vi "DAQMan TCP Data Stream.vi"() -> ()   [LabVIEW 2012]
uses:
  <userlib>/STM/_SubVIs/stm_MetaDataElement.ctl
  <userlib>/STM/TCP/stm_TCP Read Options.ctl
  Common/Controls/Waveform Header.ctl
  Common/Controls/Modified Waveform.ctl
  <userlib>/STM/TCP/STM Read Meta Data (TCP Ref).vi
  <userlib>/STM/TCP/STM Get Connection Reference (TCP).vi
  <userlib>/STM/TCP/STM Read Message (TCP).vi
panel:
  in  "Tab Control":enum32{"Wfm", "Modbus Wfm"}(tab)
  out "Acquired Data":sgl[][](graph)
  out "BlockID":u32
  out "size(s)":i32[](array[numeric])
  out "attributes (str)":string[][](array[string])
  out "Hdr Update Time":timestamp
  out "Acquired Data 2":sgl[][](graph)
  out "size(s) 2":i32[](array[numeric])
  out "BlockID 2":u32
  out "Hdr Update Time":timestamp
  out "attributes (str) 2":string[][](array[string])
  in  "Port":u16=5556
  in  "Name":T1="cDAQ1"
  out "Meta data":T1[](array[typedef])
  out "Updates":i32=2
  in  "client stop":bool
  in  "Target IP Address":string="localhost"
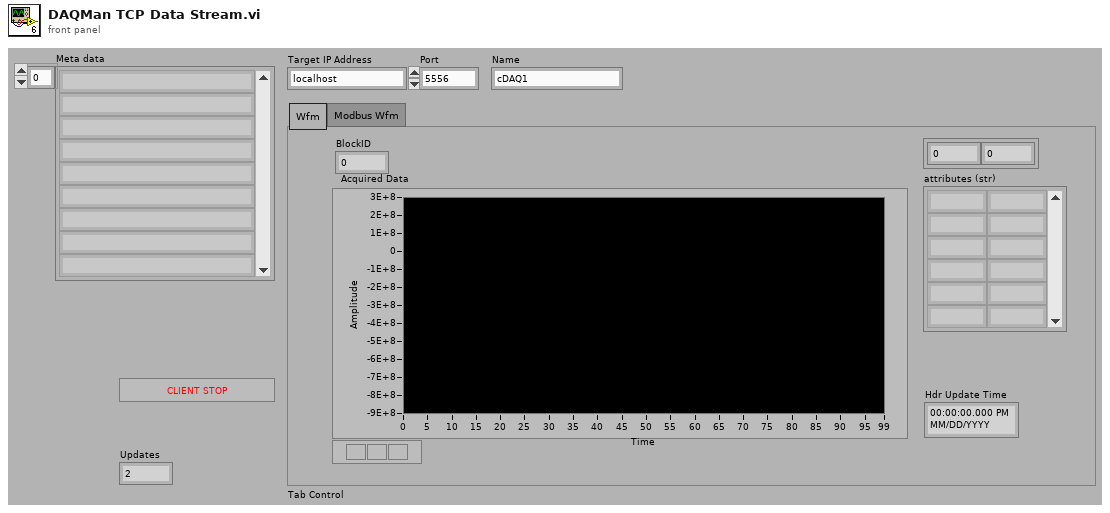
[diagram p1: front panel]
types:
  T1 = typedef "stm_MetaDataElement.ctl" = string
  T2 = typedef "stm_TCP Connection Info.ctl" = cluster{"connection ID":refnum<k5>, "Meta data":T1[]}
  T3 = typedef "stm_TCP Read Options.ctl" = cluster{"Ignore Timeout Error":bool, "timeout ms (1000)":i32}
  T4 = typedef "Waveform Header.ctl" = cluster{"dt":dbl, "attributes (str)":string[][]}
  T5 = enum16{"big-endian, network order", "native, host order", "little-endian"}
  T6 = typedef "Modified Waveform.ctl" = cluster{"BlockID":u32, "to (s)":dbl, "Y":sgl[][]}
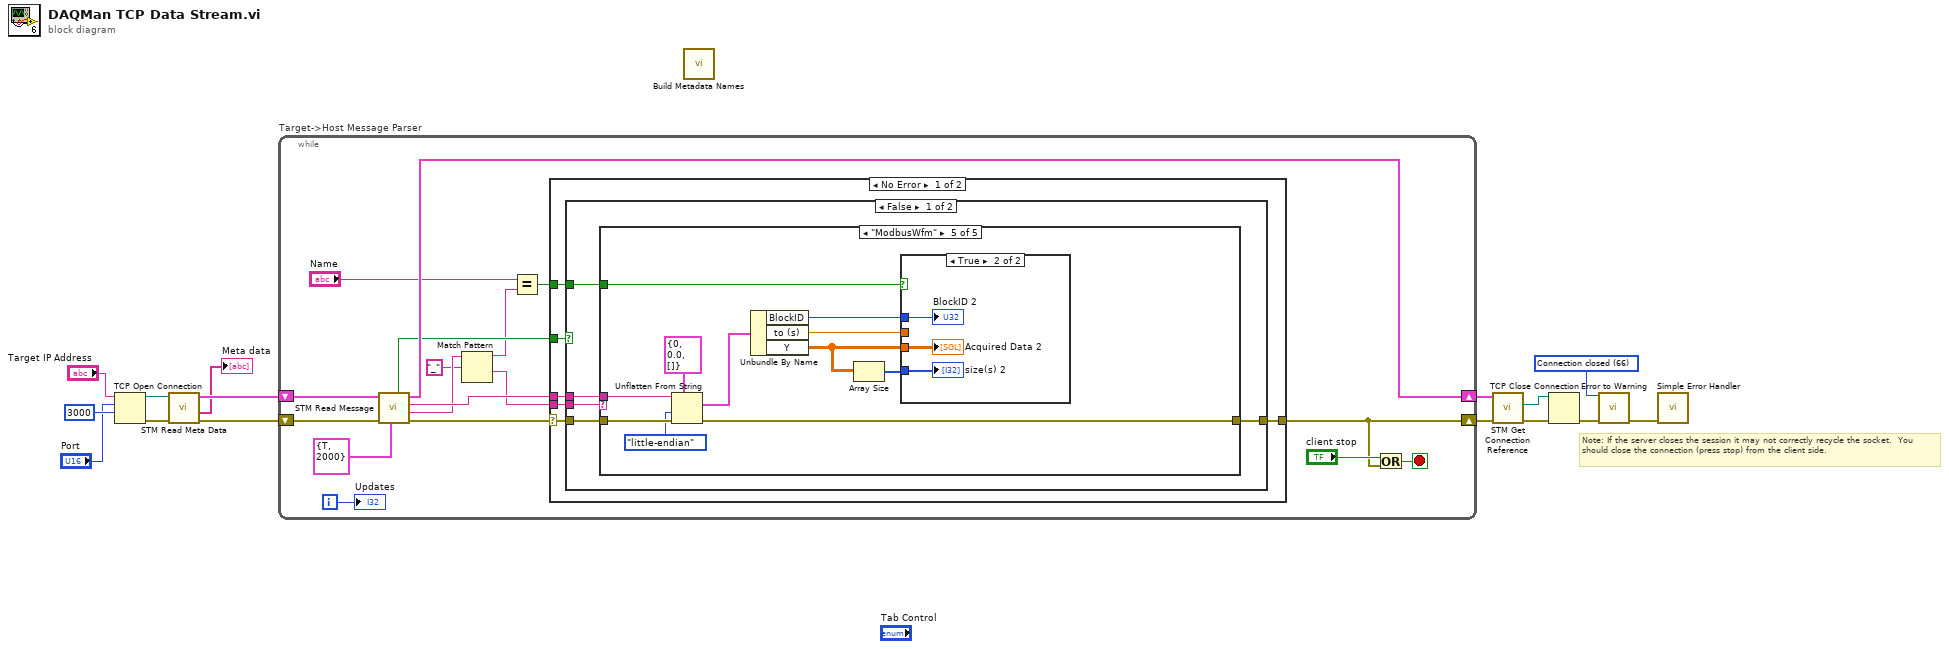
[diagram p0: block diagram]
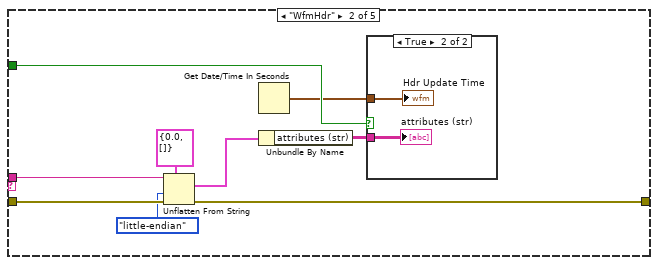
[diagram p3: hidden frame]
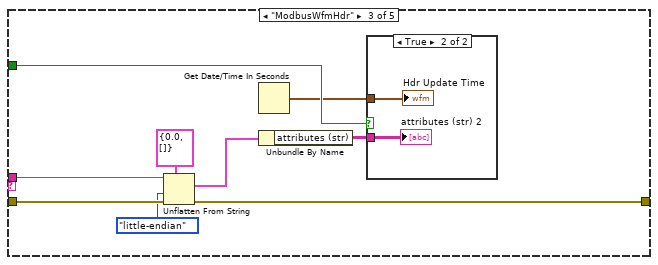
[diagram p5: hidden frame]
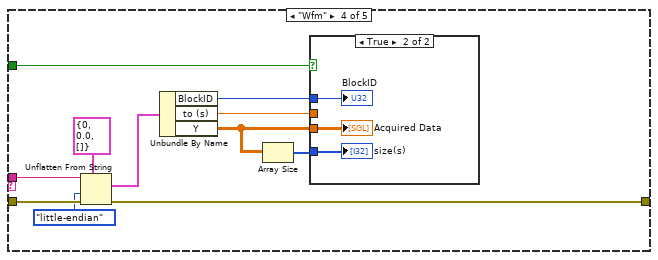
[diagram p7: hidden frame]
diagram:
  w12 = 66 items=["No Error", "Argument Error", "Memory Full", "Out of Zone", "End of File", "File Already Open", "Generic File IO Error", "File Not Found", "File Permission Error", "Disk Full", "Duplicate Path", "Too Many Files Open", "Not Enabled", "Resource File Not Found", "Cannot Add Resource", "Resource Not Found", "Image Not Found", "Image Memory Error", "Pen Does Not Exist", "Config Bad Type", "Config Token Not Found", "Config Parse Error", "Config Memory Error", "Bad External Code Format", "Bad External Code Offset", "External Code Not Present", "Null Window", "Destroy Window Mixup", "Null Menu", "Print Aborted", "Bad Print Record", "Print Driver Error", "Windows Error During Print", "Memory Error During Print", "Print Dialog Error", "Generic Print Error", "Invalid Device Refnum", "Device Not Found", "Device Parameter Error", "Device Unit Error", "Can't Open Device", "Device Call Aborted", "Generic Error", "Cancelled By User", "Object ID Too Low", "Object ID Too High", "Object Not In Heap", "Unknown Heap", "Bad DefProc ID", "DefProc Not In Table", "Message Out Of Range", "Null Method", "Unknown Message", "Manager Call Not Supported", "Bad address", "Connection In progress", "Connection timed out", "Connection is already in progress", "Network attribute not supported", "Network error", "Address in use", "System out of memory", "Connection aborted", "Connection refused", "Connection is not connected", "Connection is already connected", "Connection closed", "Initialize error (interapplication manager)", "Bad occurrence", "Wait on unbound occurrence handler", "Occurrence queue overflow", "Bad path", "Semaphore not signaled", "Unrecognized type (interapplication manager)"] ("1st Error to Convert")
  # "Note: If the server closes the session it may not correctly recycle the socket.  You should close the connection (press stop) from the client side."
  n1 = TCP Open Connection(address="Target IP Address", remote port or service name="Port", timeout ms (60000)=3000) -> (connection ID=w15:refnum<k5>, error out=w14:errorcluster)  [unwired: 1 in, 1 out]
  n2 = call-poly <userlib>:"STM Read Meta Data.vi"("error in"=w14, "connection ID"=w15) -> ("error out"=w7:errorcluster, "Meta data"=→"Meta data":T1[], "Connection Info Out"=w6:T2)  [unwired: 1 in, 6 out]
  n3 = while "Target->Host Message Parser" {
    shift-right: [w30] -> w11
    shift-left: w6 -> [w32]
    shift-right: [w22] -> w1
    shift-left: w7 -> [w31]
    i -> [w26]
    stop <- w24 stop-if-true
    n4 = call-poly <userlib>:"STM Read Message.vi"("Options"=T3 {"Ignore Timeout Error"=TRUE, "timeout ms (1000)"=2000}, "error in"=w31, "Connection Info"=w32) -> ("error out"=w27:errorcluster, "Name"=w21:T1, "data string"=w29:string, "Connection Info Out"=w30:T2, "Timed Out?"=w28:bool)  [unwired: 2 in, 2 out]
    n5 = Match Pattern(string=w21, regular expression="_") -> (before substring=w18:T1, after substring=w20:T1)  [unwired: 1 in, 2 out]
    n6 = Equal?(x="Name", y=w18) -> (x = y?=w16:bool)
    n7 = case shown="No Error" w27 {
      selector: w27 -> [w36 w96]
      tunnel: w29 -> [w38 _]
      tunnel: w28 -> [w37 _]
      tunnel: [w35 w96] -> w22
      tunnel: w20 -> [w34 _]
      tunnel: w16 -> [w33 _]
      frame No Error {
        n8 = case shown="False" w37 {
          tunnel: w38 -> [w43 _]
          tunnel: w36 -> [w42 w95]
          tunnel: [w41 w95] -> w35
          tunnel: w34 -> [w40 _]
          tunnel: w33 -> [w39 _]
          frame False {
            n9 = case shown="\"ModbusWfm\"" w40 {
              tunnel: w43 -> [_ w53 w64 w77 w91]
              tunnel: w42 -> [w44 w52 w63 w76 w90]
              tunnel: [w44 w51 w62 w75 w89] -> w41
              tunnel: w39 -> [_ w46 w57 w68 w82]
              frame Default {
              }
              frame "WfmHdr" {
                n10 = Unflatten From String(type=T4 {"dt"=0.0, "attributes (str)"=[]} ("Wfm Header"), binary string=w53, byte order (0:big-endian, network order)=T5."little-endian", error in (no error)=w52) -> (value=w48:T4, error out=w51:errorcluster)  [unwired: 2 out]
                n11 = Get Date/Time In Seconds() -> (seconds since 1Jan1904=w45:timestamp)
                n12 = Unbundle By Name(w48) -> ("attributes (str)"=w47:string[][])
                n13 = case shown="True" w46 {
                  tunnel: w47 -> [_ w55]
                  tunnel: w45 -> [_ w54]
                  frame False {
                  }
                  frame True {
                    "attributes (str)" <- w55
                    "Hdr Update Time" <- w54
                  }
                }
              }
              frame "ModbusWfmHdr" {
                n14 = Unflatten From String(type=T4 {"dt"=0.0, "attributes (str)"=[]} ("Wfm Header"), binary string=w64, byte order (0:big-endian, network order)=T5."little-endian", error in (no error)=w63) -> (value=w59:T4, error out=w62:errorcluster)  [unwired: 2 out]
                n15 = Get Date/Time In Seconds() -> (seconds since 1Jan1904=w56:timestamp)
                n16 = Unbundle By Name(w59) -> ("attributes (str)"=w58:string[][])
                n17 = case shown="True" w57 {
                  tunnel: w58 -> [_ w66]
                  tunnel: w56 -> [_ w65]
                  frame False {
                  }
                  frame True {
                    "attributes (str) 2" <- w66
                    "Hdr Update Time" <- w65
                  }
                }
              }
              frame "Wfm" {
                n18 = Unflatten From String(type=T6 {"BlockID"=0, "to (s)"=0.0, "Y"=[]} ("Modified Waveform"), binary string=w77, byte order (0:big-endian, network order)=T5."little-endian", error in (no error)=w76) -> (value=w74:T6, error out=w75:errorcluster)  [unwired: 2 out]
                n19 = Unbundle By Name(w74) -> ("BlockID"=w73:u32, "to (s)"=w67:dbl, "Y"=w70:sgl[][])
                n20 = Array Size(array=w70) -> (size(s)=w69:i32[])
                n21 = case shown="True" w68 {
                  tunnel: w73 -> [_ w80]
                  tunnel: w70 -> [_ w79]
                  tunnel: w69 -> [_ w78]
                  tunnel: w67 -> [_ _]
                  frame False {
                  }
                  frame True {
                    "Acquired Data" <- w79
                    "BlockID" <- w80
                    "size(s)" <- w78
                  }
                }
              }
              frame "ModbusWfm" {
                n22 = Unflatten From String(type=T6 {"BlockID"=0, "to (s)"=0.0, "Y"=[]} ("Modified Waveform"), binary string=w91, byte order (0:big-endian, network order)=T5."little-endian", error in (no error)=w90) -> (value=w88:T6, error out=w89:errorcluster)  [unwired: 2 out]
                n23 = Unbundle By Name(w88) -> ("BlockID"=w87:u32, "to (s)"=w81:dbl, "Y"=w84:sgl[][])
                n24 = Array Size(array=w84) -> (size(s)=w83:i32[])
                n25 = case shown="True" w82 {
                  tunnel: w87 -> [_ w94]
                  tunnel: w84 -> [_ w93]
                  tunnel: w83 -> [_ w92]
                  tunnel: w81 -> [_ _]
                  frame False {
                  }
                  frame True {
                    "Acquired Data 2" <- w93
                    "BlockID 2" <- w94
                    "size(s) 2" <- w92
                  }
                }
              }
            }
          }
          frame True {
          }
        }
      }
      frame Error {
      }
    }
    n26 = Or(x="client stop", y=w22) -> (x .or. y?=w24:bool)
    "Updates" <- w26
  }
  n27 = call "Build Metadata Names.vi"() -> ()  [unwired: 7 in, 5 out]
  n28 = call-poly <userlib>:"STM Get Connection Reference.vi"("error in"=w1, "Connection Info"=w11) -> ("error out"=w9:errorcluster, "connection ID out"=w10:refnum<k5>)  [unwired: 8 out]
  n29 = TCP Close Connection(connection ID=w10, error in (no error)=w9) -> (error out=w8:errorcluster)  [unwired: 2 out]
  n30 = call <vilib>:"Error to Warning.vi"("1st Error to Convert"=w12, "error in"=w8) -> ("warning out"=w5:errorcluster)  [unwired: 3 in, 10 out]
  n31 = call <vilib>:"Simple Error Handler.vi"("error in (no error)"=w5) -> ()  [unwired: 4 in, 5 out]
